vi "Filter by Class.vi"(8 "error in (no error)":errorcluster, 10 "Filter":string, 11 "Shapes in":refnum<data-value>[](array[refnum])) -> (0 "error out":errorcluster, 3 "Shapes out":refnum<data-value>[](array[refnum]))   [LabVIEW 2017, in "LV Image Editor Framework.lvlib" / "Image Editor Handler.lvclass"]
uses:
  Image Editor Handler.lvclass
  Forms/Shape/Shape.lvclass
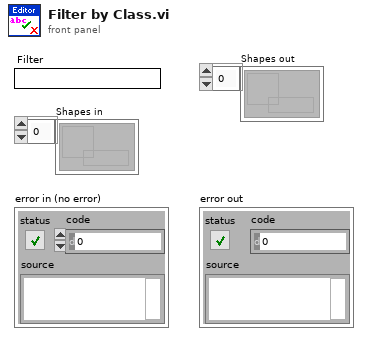
[diagram p1: front panel]
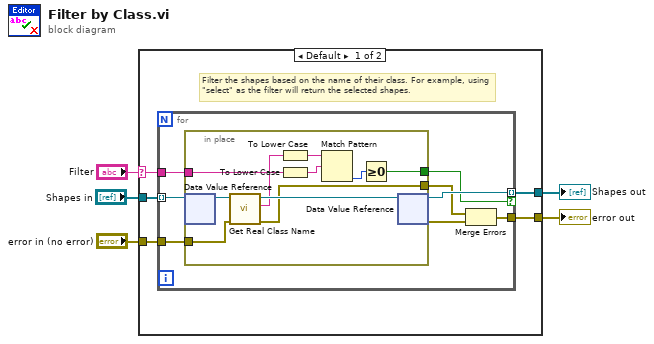
[diagram p0: block diagram]
diagram:
  n1 = case shown="Default" "Filter" {
    selector: "Filter" -> [w9 _]
    tunnel: "Shapes in" -> [w10 w30]
    tunnel: [w8 w30] -> w3
    tunnel: "error in (no error)" -> [w7 w29]
    tunnel: [w6 w29] -> w5
    frame Default {
      # "Filter the shapes based on the name of their class. For example, using \"select\" as the filter will return the selected shapes."
      n2 = for {
        tunnel: w10 -> [w18] mode=indexing
        tunnel: w9 -> [w17]
        tunnel: [w16] -> w8 mode=indexing if=w15
        tunnel: w7 -> [w14]
        tunnel: [w12] -> w6
        n3 = in-place {
          in-place-border: w17 -> [w28]
          in-place-border: [w26] -> w15
          in-place-border: w14 -> [w19]
          in-place-border: [w20] -> w11
          n4 = in-place-dvr #1(w18) -> (w23:refnum<class "Shape.lvclass">)  [unwired: 1 out]
          n5 = call-dynamic "Get Real Class Name.vi"("error in (no error)"=w19, "Shape in"=w23) -> ("error out"=w20:errorcluster, "Real Class"=w21:string, "Shape out"=w22:refnum<class "Shape.lvclass">)  [unwired: 7 in]
          n6 = To Lower Case(string=w21) -> (all lower case string=w24:string)
          n7 = To Lower Case(string=w28) -> (all lower case string=w25:string)
          n8 = Match Pattern(string=w24, regular expression=w25) -> (offset past match=w27:i32)  [unwired: 1 in, 3 out]
          n9 = Greater Or Equal To 0?(x=w27) -> (x >= 0?=w26:bool)
          n10 = in-place-dvr #1(w22) -> (w16:refnum<data-value>, w13:errorcluster)
        }
        n11 = Merge Errors(w11, w13) -> (w12:errorcluster)
      }
    }
    frame "" {
      # "Empty string: don't filter and return all the shapes in the picture"
    }
  }
  "error out" <- w5
  "Shapes out" <- w3
